vi "Function.Handle Default Case.vi"(5 "Timeout(s)":dbl, 6 "Other Modules":string[](array[string]), 7 "Child Modules":cluster{"Name":string, "vi ref":refnum<vi>}[](array[cluster]), 8 "Error In":errorcluster, 9 "Data1 In":variant, 10 "Funct Name":string, 11 "Q In":refnum<queue>) -> (0 "RTN Error":errorcluster, 3 "RTN Vars":string[][](array[string]))   [LabVIEW 2019]
uses:
  <vilib>/KATE/Queues/Q.Element.ctl
  Errors/Error.Error Code List.ctl
  <vilib>/KATE/Queues/Queue Utils.lvlib
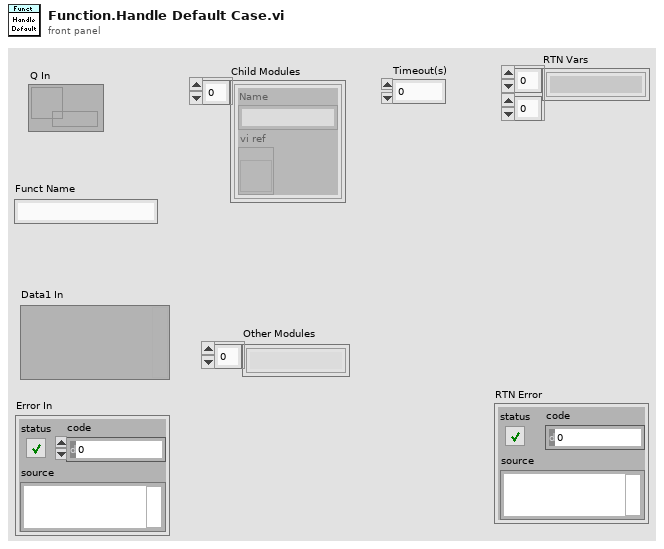
[diagram p1: front panel]
types:
  T1 = typedef "Error.Error Code List.ctl" = i32
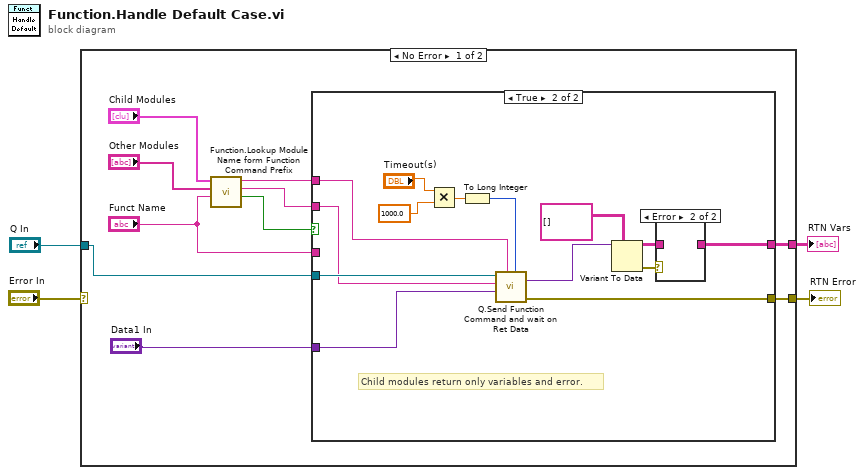
[diagram p0: block diagram]
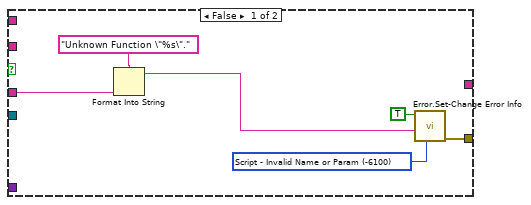
[diagram p2: hidden frame]
diagram:
  n1 = case shown="No Error" "Error In" {
    selector: "Error In" -> [_ w36]
    tunnel: [w14 _] -> w4
    tunnel: [w13 w36] -> w3
    tunnel: "Q In" -> [w5 _]
    frame No Error {
      n2 = call "Function.Lookup Module Name form Function Command Prefix.vi"("Function Name with Prefix"="Funct Name", "Other Modules"="Other Modules", "Child Modules"="Child Modules") -> ("Found"=w9:bool, "Function Name"=w7:string, "Module Name"=w8:string)  [unwired: 6 in]
      n3 = case shown="True" w9 {
        tunnel: [w19 w29] -> w13
        tunnel: w5 -> [_ w31]
        tunnel: "Data1 In" -> [_ w30]
        tunnel: [_ w24] -> w14
        tunnel: w8 -> [_ w22]
        tunnel: w7 -> [_ w21]
        tunnel: "Funct Name" -> [w15 _]
        frame False {
          w18 = T1 -6100 items=["No Error"=0, "Abort"=-2, "Misc"=-5000, "Fixture Error"=-5100, "File IO - General"=-5200, "FIle IO - Config Error"=-5201, "Instrument - General"=-5300, "Instrument - Serial Com"=-5301, "Instrument - Camera"=-5302, "Instrument - PS"=-5303, "Instrument - Oscilloscope"=-5304, "Instrument - Function Gen"=-5305, "Instrument - Load"=-5306, "Instrument - Meter"=-5307, "Instrument - Power Control"=-5308, "Instrument - Motion"=-5309, "Instrument - RF"=-5310, "System Exe"=-5400, "Image Processing"=-5500, "Communication"=-5600, "Script - Syntax Error"=-6000, "Script - Invalid Name or Param"=-6100, "Script - Timeout"=-6200, "Invalid Data"=-6300, "FW Update Error"=-6500] ("Std Code")
          n4 = Format Into String(format string="Unknown Function \"%s\".", w15) -> (resulting string=w16:string)  [unwired: 2 in, 1 out]
          n5 = call "Error.Set-Change Error Info.vi"("Std Code"=w18, "Description"=w16, "Set Error"=TRUE) -> ("error out"=w19:errorcluster)  [unwired: 8 in]
        }
        frame True {
          # "Child modules return only variables and error."
          n6 = Multiply(x="Timeout(s)", y=1000.0) -> (x*y=w33:dbl)
          n7 = To Long Integer(number=w33) -> (32bit integer=w32:i32)
          n8 = call <vilib>:"Q.Send Function Command and wait on Ret Data.vi"("Timeout(ms)"=w32, "Q Name"=w22, "Data1"=w30, "Cmd"=w21, "Q In"=w31) -> ("error out"=w29:errorcluster, "Ret"=w25:variant)  [unwired: 5 in]
          n9 = Variant To Data(type=string[][] [], Variant=w25) -> (data=w26:string[][], error out=w27:errorcluster)  [unwired: 1 in]
          n10 = case shown="Error" w27 {
            tunnel: w26 -> [w35 _]
            tunnel: [w35 _] -> w24
            frame No Error {
            }
            frame Error {
            }
          }
        }
      }
    }
    frame Error {
    }
  }
  "RTN Vars" <- w4
  "RTN Error" <- w3
